vi "reset AO_galvo_stim.vi"(8 "error in (no error)":errorcluster) -> (0 "error out":errorcluster)   [LabVIEW 2012]
doc: "SciScan 1.0 151216"
uses:
  <vilib>/DAQmx/write.llb/DAQmx Write.vi
  <vilib>/DAQmx/write.llb/DAQmx Write (Analog 1D DBL NChan 1Samp).vi
  GFG/GFGstringGet.vi
  <vilib>/DAQmx/create/channels.llb/DAQmx Create Channel (AO-Voltage-Basic).vi
  <vilib>/DAQmx/miscellaneous.llb/DAQmx Fill In Error Info.vi
  GFG/GFG library.lvlib
panel:
  out "error out 2":errorcluster
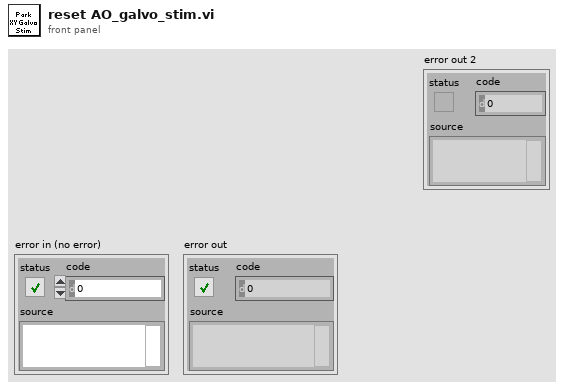
[diagram p1: front panel]
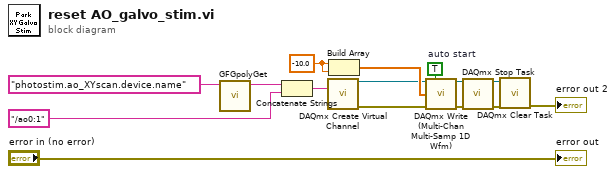
[diagram p0: block diagram]
diagram:
  w9 = TRUE  # auto start
  w6 = -10.0 ("data")
  n1 = call-poly "GFGpolyGet.vi"("Variable Name in"="photostim.ao_XYscan.device.name") -> ("String"=w2:string)  [unwired: 9 in, 1 out]
  n2 = Concatenate Strings(w2, "/ao0:1" ("string")) -> (w1:string)
  n3 = call-poly <vilib>:"DAQmx Create Virtual Channel.vi"("physical channels"=w1) -> ("task out"=w8:refnum<k21>, "error out"=w10:errorcluster)  [unwired: 13 in]
  n4 = Build Array(w6, w6) -> (w15:dbl[])
  n5 = call-poly "DAQmx Write (Multi-Chan Multi-Samp 1D Wfm).vi"("task/channels in"=w8, "auto start"=w9, "data"=w15, "error in"=w10) -> ("task out"=w7:refnum<k21>, "error out"=w11:errorcluster)  [unwired: 9 in, 1 out]
  n6 = call <vilib>:"DAQmx Stop Task.vi"("task/channels in"=w7, "error in"=w11) -> ("task out"=w13:refnum<k21>, "error out"=w12:errorcluster)  [unwired: 12 in]
  n7 = call <vilib>:"DAQmx Clear Task.vi"("task in"=w13, "error in"=w12) -> ("error out"=→"error out 2":errorcluster)  [unwired: 13 in]
  "error out" <- "error in (no error)"
